vi "ASI_z_control onoff.vi"(2 "Z control":bool, 3 "error in (no error)":errorcluster, 4 "Method":u16(ring) items=["Analogue", "Serial"], 5 "VISA resource name":refnum<visa-resource-name>) -> (0 "error out":errorcluster, 1 "VISA resource name out":refnum<visa-resource-name>)   [LabVIEW 2012]
panel:
  out "Serial Settings:Number of Bytes at Serial Port":u32
  out "read buffer":string
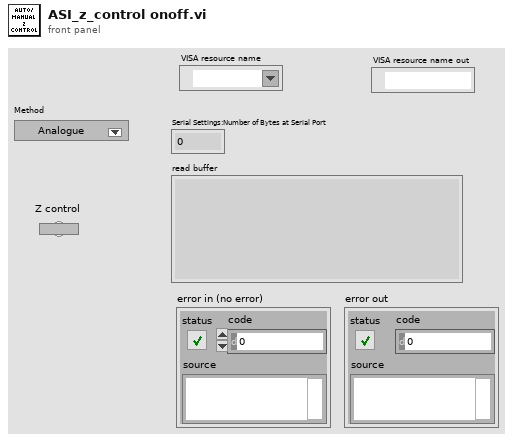
[diagram p1: front panel]
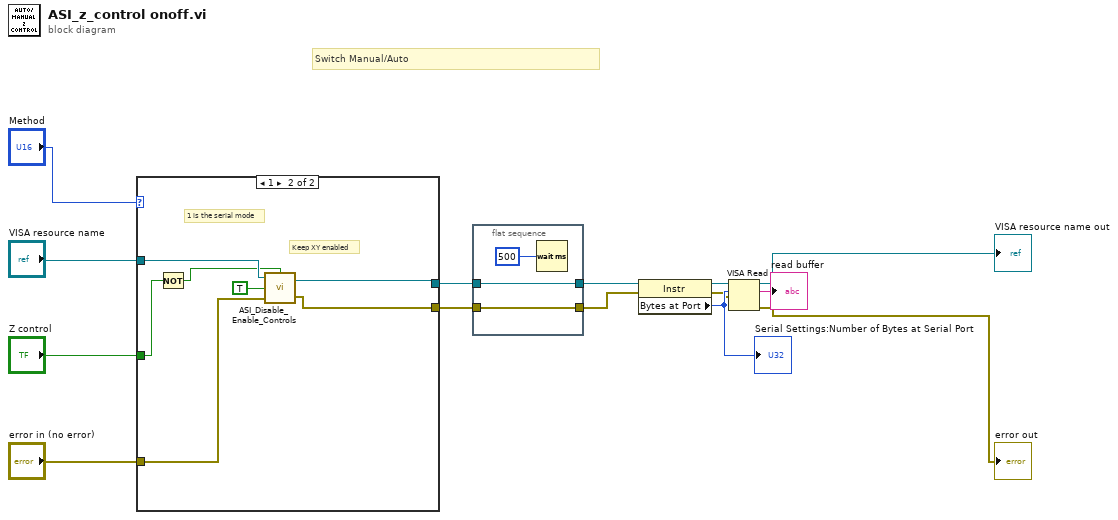
[diagram p0: block diagram]
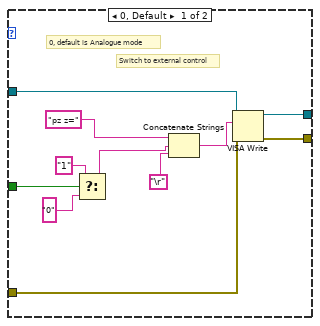
[diagram p2: hidden frame]
diagram:
  # "Switch Manual/Auto"
  n1 = case shown="1" "Method" {
    tunnel: "Z control" -> [w19 w27]
    tunnel: [w18 w29] -> w9
    tunnel: "VISA resource name" -> [w17 w31]
    tunnel: "error in (no error)" -> [w16 w32]
    tunnel: [w15 w28] -> w4
    frame 0, Default {
      # "Switch to external control"
      # "0, default is Analogue mode"
      n2 = Select(t="1", s=w19, f="0") -> (s? t:f=w21:string)
      n3 = Concatenate Strings("pz z=", w21, "\r") -> (w20:string)
      n4 = VISA Write(VISA resource name=w17, write buffer=w20, error in (no error)=w16) -> (VISA resource name out=w18:refnum<visa-resource-name>, error out=w15:errorcluster)  [unwired: 1 out]
    }
    frame 1 {
      # "Keep XY enabled"
      # "1 is the serial mode"
      n5 = Not(x=w27) -> (.not. x?=w26:bool)
      n6 = call "ASI_Disable_Enable_Controls.vi"("Disable Z"=w26, "error in"=w32, "Disable XY"=TRUE, "VISA resource name"=w31) -> ("error out"=w28:errorcluster, "VISA resource name out"=w29:refnum<visa-resource-name>)
    }
  }
  n7 = flat-sequence {
    tunnel: [w35] -> w10
    tunnel: w9 -> [w35]
    tunnel: [w33] -> w5
    tunnel: w4 -> [w33]
    frame #0 {
      n8 = Wait (ms)(milliseconds to wait=u32 500) -> ()  [unwired: 1 out]
    }
  }
  n9 = property class="Instr"(reference=w10, error in=w5) -> (reference out=w13:refnum<visa-resource-name>, error out=w3:errorcluster, "Bytes at Port"=w12:u32)
  "Serial Settings:Number of Bytes at Serial Port" <- w12
  n10 = VISA Read(VISA resource name=w13, byte count=w12, error in (no error)=w3) -> (VISA resource name out=→"VISA resource name out":refnum<visa-resource-name>, read buffer=→"read buffer":string, error out=→"error out":errorcluster)  [unwired: 1 out]
